vi "Dynamic Dispatch.Static.vi"() -> ()   [LabVIEW 2016]
uses:
  <vilib>/Platform/TimedLoop/XDataNode/timing_clust.ctl
  <vilib>/Platform/TimedLoop/XDataNode/nitl_modes.ctl
  <vilib>/Platform/TimedLoop/XDataNode/wakeup.ctl
  Classes/Child A/DD Child A.lvclass
  <vilib>/platform/TimedLoop/XDataNode/XDataNode.xnode
  <vilib>/Platform/TimedLoop/XDataNode/XDNodeRunTimeDep.lvlib
panel:
  out "first iteration":u32
  in  "Iterations":i32=1000
  out "durations":u32[](graph)
  in  "processor":i32=-2
  out "name":string
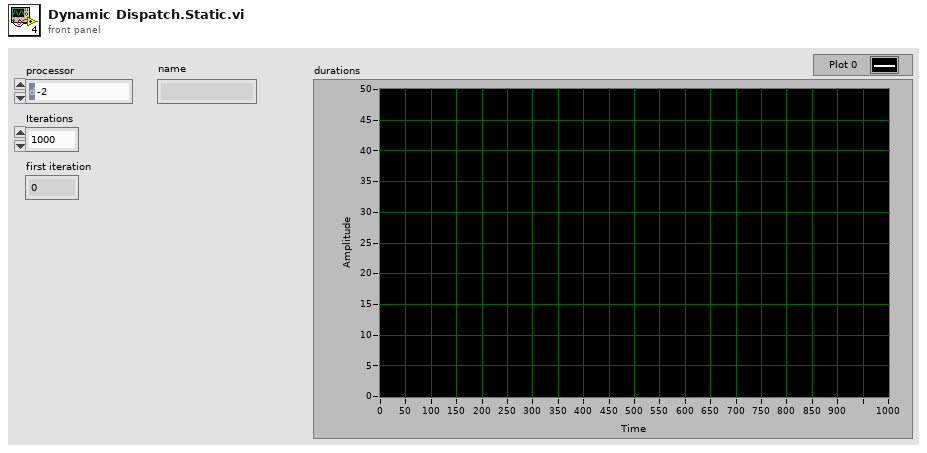
[diagram p1: front panel]
types:
  T1 = typedef "XDNodeRunTimeDep.lvlib/timing_clust.ctl" = cluster{"Expected End [f-1]":u64, "Actual End [f-1]":u64, "Finished Late? [f-1]":bool, "Expected End [i-1]":u64, "Actual End [i-1]":u64, "Finished Late? [i-1]":bool, "Expected Start [i]":u64, "Actual Start [i]":u64, "Expected Start [f]":u64, "Actual Start [f]":u64, "Source Name":string, "Structure Name":string, "Period":i64, "Deadline":i64, "Offset":i64, "Start":i64, "Priority":i32, "Timeout":i32, "Mode":T2, "Wakeup Reason":T3, "Error":errorcluster, "Source Type":string, "Secondary Source Type":string, "Global End Time":u64, "Global Start Time":u64, "Frame Duration":u64, "Iteration Duration":u64, "Assigned CPU":i32, "I/O Scan Engine Mode":u32}
  T2 = typedef "XDNodeRunTimeDep.lvlib/nitl_modes.ctl" = enum32{"No Change", "Process missed periods, maintain original phase", "Discard missed periods, maintain original phase", "Process missed periods, ignore original phase", "Discard missed periods, ignore original phase"}
  T3 = typedef "XDNodeRunTimeDep.lvlib/wakeup.ctl" = enum32{"Normal", "Aborted", "Asynchronous wakeup", "Timing source error", "Timed loop error", "Timeout"}
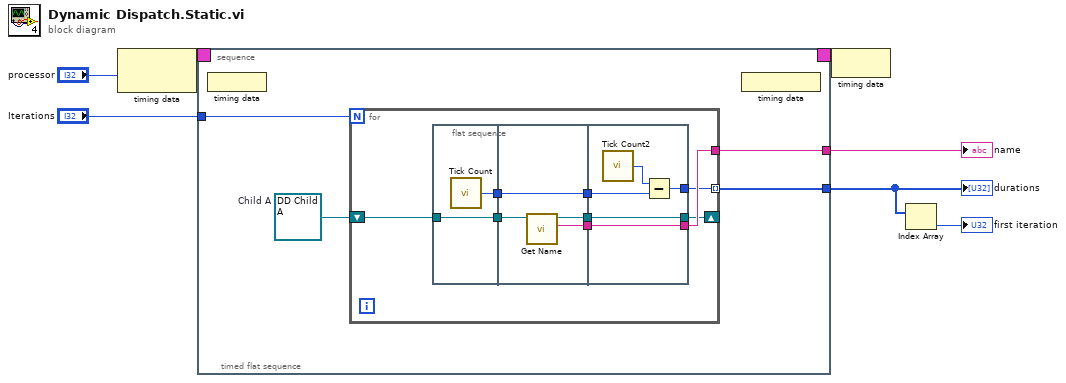
[diagram p0: block diagram]
diagram:
  n1 = node-c288("processor") -> (w7:T1)
  n2 = timed-sequence {
    timing: w7 -> [_]
    timing-out: [_] -> w6
    tunnel: [w10] -> w4
    tunnel: [w9] -> w3
    tunnel: "Iterations" -> [w8]
    n3 = timed-flat-sequence {
      tunnel: [w14] -> w10
      tunnel: [w13] -> w9
      tunnel: w8 -> [w12]
      w11 = refnum<class "DD Child A.lvclass"> refnum  # Child A
      n4 = node-c288() -> ()  [unwired: 1 in]
      n5 = for {
        N: w12 -> [_]
        tunnel: [w21] -> w14
        tunnel: [w20] -> w13 mode=indexing
        shift-right: [w17] -> _
        shift-left: w11 -> [w18]
        n6 = flat-sequence {
          tunnel: [w27] -> w25
          tunnel: w18 -> [w26]
          tunnel: [w26] -> w19
          tunnel: [w31] -> w24
          tunnel: w25 -> [w30]
          tunnel: [w30] -> w23
          tunnel: [w29] -> w22
          tunnel: w19 -> [w28]
          tunnel: [w36] -> w21
          tunnel: w24 -> [w36]
          tunnel: w23 -> [w35]
          tunnel: [w33] -> w20
          tunnel: w22 -> [w32]
          tunnel: [w32] -> w17
          frame #0 {
            n7 = call "Tick Count"() -> ("Tick Count(uSec)"=w27:u32)
          }
          frame #1 {
            n8 = call-dynamic "Get Name.vi"("DD Child A in"=w28) -> ("name"=w31:string, "DD Child A out"=w29:refnum<class "DD Child A.lvclass">)  [unwired: 8 in, 1 out]
          }
          frame #2 {
            n9 = call "Tick Count2"() -> ("Tick Count(uSec)"=w34:u32)
            n10 = Subtract(x=w34, y=w35) -> (x-y=w33:u32)
          }
        }
      }
      n11 = node-c288() -> ()  [unwired: 1 out]
    }
  }
  "name" <- w4
  "durations" <- w3
  n12 = node-c288(w6) -> ()
  n13 = Index Array(array=w3) -> (element=→"first iteration":u32)  [unwired: 1 in]
